vi "RX.vi"() -> ()   [LabVIEW 2020]
panel:
  in  "Частота \nдискритезации":dbl=5000000.0 format="%#_13g"
  in  "Время \nнакопления":dbl=0.008 format="%#_13g"
  out "qC/N0 dB":dbl
  out "qC/N0":dbl
  out "dopEst":dbl
  out "codePhase":dbl
  in  "NKA id":dbl=1.0
  in  "Целое число строк записанного файла":i32=100
  in  "Путь к записи сигнала":path=path "C:/Users/ira_1/OneDrive/Рабочий стол/samples.bin"
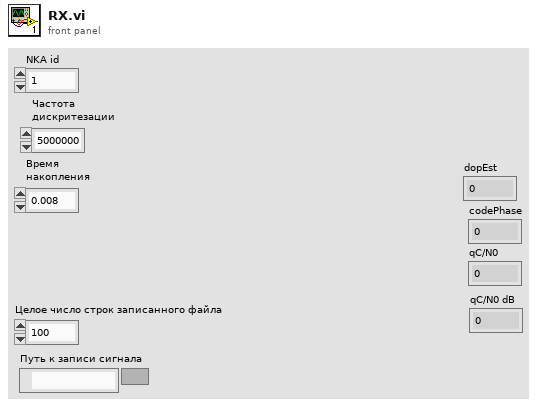
[diagram p1: front panel]
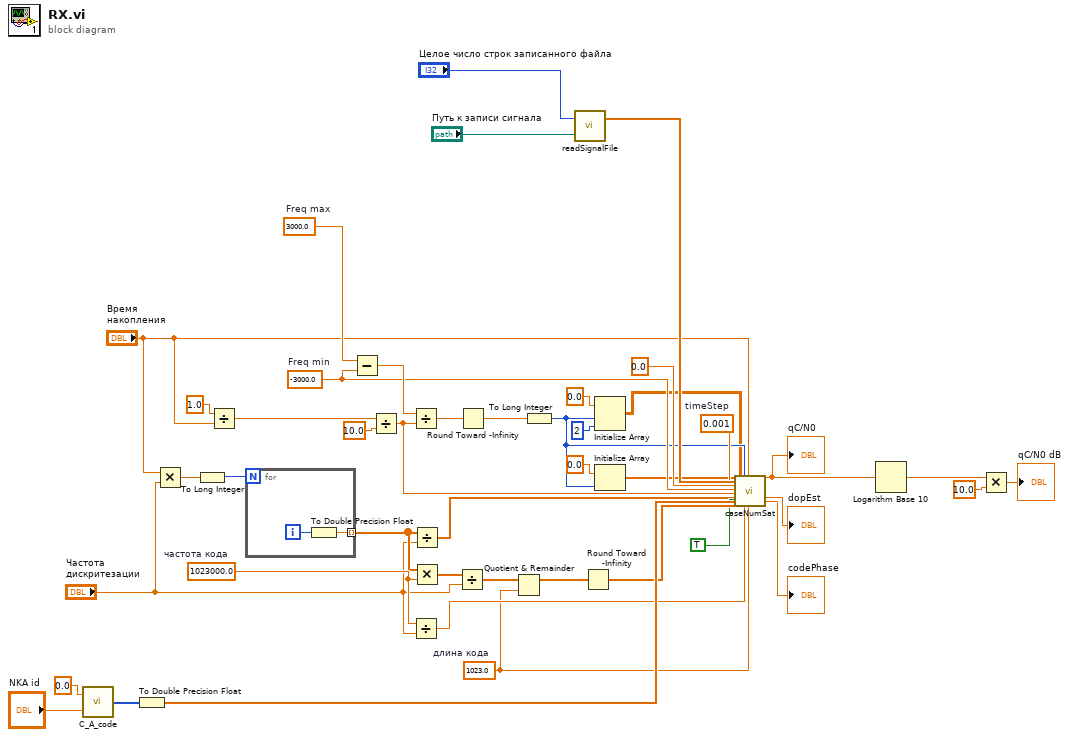
[diagram p0: block diagram]
diagram:
  w19 = 0.001  # timeStep
  w25 = -3000.0  # Freq min
  w31 = 3000.0  # Freq max
  w21 = 1023.0  # длина кода
  w23 = 1023000.0  # частота кода
  n1 = call "C_A_code.vi"("NKA id"="NKA id", "Delay"=0.0) -> ("Value"=w39:i32[])
  n2 = To Double Precision Float(number=w39) -> (double precision float=w38:dbl[])
  n3 = Multiply(x="Время \nнакопления", y="Частота \nдискритезации") -> (x*y=w1:dbl)
  n4 = To Long Integer(number=w1) -> (32bit integer=w2:i32)
  n5 = Divide(x=1.0, y="Время \nнакопления") -> (x/y=w27:dbl)
  n6 = for {
    N: w2 -> [_]
    tunnel: [w45] -> w10 mode=indexing
    i -> [w46]
    n7 = To Double Precision Float(number=w46) -> (double precision float=w45:dbl)
  }
  n8 = Subtract(x=w31, y=w25) -> (x-y=w29:dbl)
  n9 = Divide(x=w27, y=10.0) -> (x/y=w24:dbl)
  n10 = Divide(x=w29, y=w24) -> (x/y=w30:dbl)
  n11 = Divide(x=w23, y="Частота \nдискритезации") -> (x/y=w22:dbl)
  n12 = Divide(x=w10, y="Частота \nдискритезации") -> (x/y=w9:dbl[])
  n13 = Multiply(x=w10, y=w23) -> (x*y=w37:dbl[])
  n14 = Divide(x=w37, y="Частота \nдискритезации") -> (x/y=w36:dbl[])
  n15 = Round Toward -Infinity(1:w30) -> (0:w28:dbl)
  n16 = Quotient & Remainder(x=w36, y=w21) -> (x-y*floor(x/y)=w35:dbl[])  [unwired: 1 out]
  n17 = To Long Integer(number=w28) -> (32bit integer=w15:i32)
  n18 = call "readSignalFile.vi"("Путь к записи сигнала"="Путь к записи сигнала", "Целое число строк записанного файла"="Целое число строк записанного файла") -> ("subarray"=w43:cdb[])  [unwired: 1 out]
  n19 = Round Toward -Infinity(1:w35) -> (0:w34:dbl[])
  n20 = Initialize Array(0.0 ("element"), w15, 2 ("dimension size")) -> (w14:dbl[][])
  n21 = Initialize Array(0.0 ("element"), w15) -> (w13:dbl[])
  n22 = call "caseNumSat.vi"("emptyVarCorrArr"=w13, "signalArrCDB"=w43, "iFreq"=0.0, "Freq min"=w25, "Freq cell"=w24, "SampTimeArr"=w9, "PSPcodeL1C/A"=w38, "PSPcodeL1C/AIndex"=w34, "emptyCorrArr"=w14, "numCellFreq"=w15, "codeFreqDivAdcFreq"=w22, "timeAccumAcq"="Время \nнакопления", "codeLength"=w21, "timeStep"=w19, "isThisNumTry"=TRUE) -> ("cn0Est"=w6:dbl, "dopEst"=→"dopEst":dbl, "codePhase"=→"codePhase":dbl)  [unwired: 6 in, 4 out]
  "qC/N0" <- w6
  n23 = Logarithm Base 10(1:w6) -> (0:w8:dbl)
  n24 = Multiply(x=w8, y=10.0) -> (x*y=→"qC/N0 dB":dbl)
